vi "Program20.vi"() -> ()   [LabVIEW 2020]
panel:
  out "Array":dbl[][](array[numeric])
  out "initialized array":dbl[][](array[numeric])
  out "Rozmiar tablicy":i32[](array[numeric])
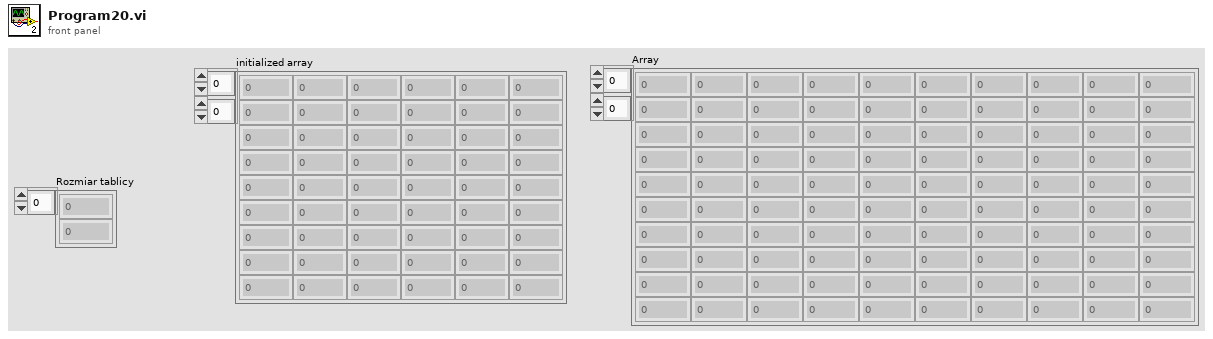
[diagram p1: front panel]
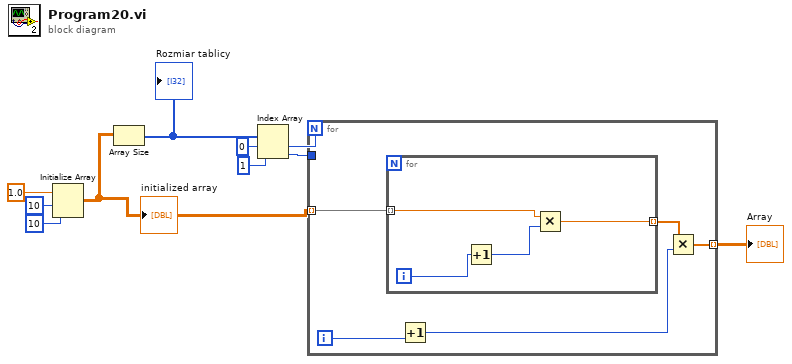
[diagram p0: block diagram]
diagram:
  n1 = Initialize Array(1.0 ("element"), 10 ("dimension size"), 10 ("dimension size")) -> (w2:dbl[][])
  "initialized array" <- w2
  n2 = Array Size(array=w2) -> (size(s)=w8:i32[])
  "Rozmiar tablicy" <- w8
  n3 = Index Array(array=w8, index #1=0 ("index"), index #2=1 ("index")) -> (element #1=w4:i32, element #2=w3:i32)
  n4 = for {
    N: w4 -> [_]
    tunnel: w3 -> [_]
    tunnel: [w15] -> w1 mode=indexing
    tunnel: w2 -> [w11] mode=indexing
    i -> [w13]
    n5 = for {
      tunnel: [w19] -> w14 mode=indexing
      tunnel: w11 -> [w16] mode=indexing
      i -> [w17]
      n6 = Increment(x=w17) -> (x+1=w18:i32)
      n7 = Multiply(x=w16, y=w18) -> (x*y=w19:dbl)
    }
    n8 = Increment(x=w13) -> (x+1=w12:i32)
    n9 = Multiply(x=w14, y=w12) -> (x*y=w15:dbl[])
  }
  "Array" <- w1
